vi "test-new-clock64-benchmark.vi"() -> ()   [LabVIEW 2020]
uses:
  <vilib>/Rock Robotics/WPI/ThirdParty/JAS_Junk/TrajLib/VI/Util_GetTime_U32.vi
  <vilib>/Rock Robotics/SystemInterfaces/Utilities/FPGA_UtilitiesRead LocalTime.vi
  <vilib>/Rock Robotics/WPI/ThirdParty/JAS_Junk/TrajLib/Trajectory_Library.lvlib
panel:
  out "Avg Loop US":dbl
  out "Per Loop US":dbl
  out "Error Count":i32
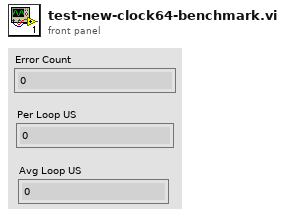
[diagram p1: front panel]
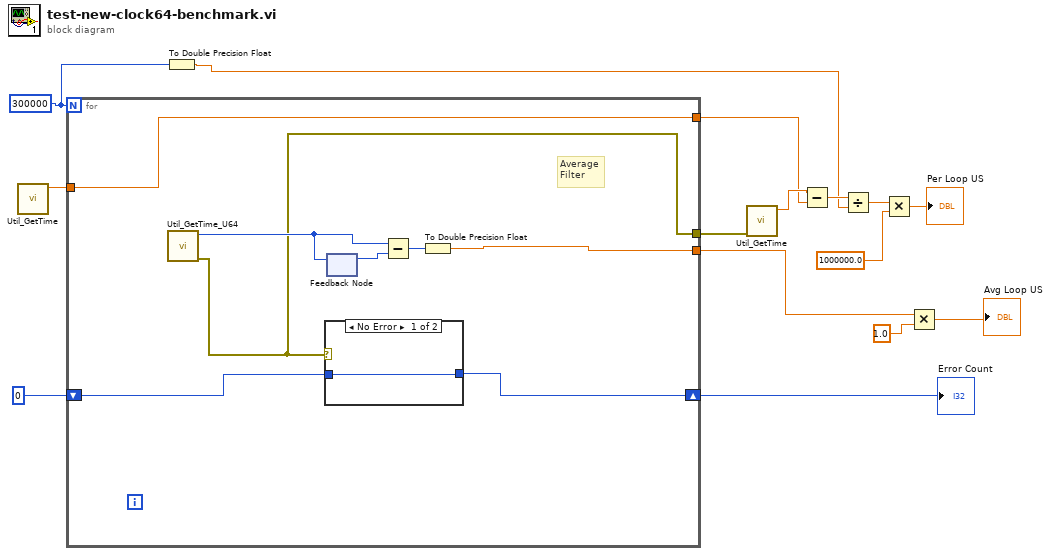
[diagram p0: block diagram]
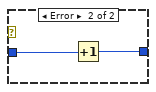
[diagram p2: hidden frame]
diagram:
  w13 = 300000
  n1 = call <vilib>:"Util_GetTime.vi"() -> ("FPGA_Time_Seconds"=w15:dbl)  [unwired: 8 in, 3 out]
  n2 = for {
    N: w13 -> [_]
    tunnel: w15 -> [w20]
    shift-right: [w21] -> w9
    shift-left: 0 -> [w23]
    tunnel: [w16] -> w4
    tunnel: [w20] -> w6
    tunnel: [w17] -> w2
    # "Average\nFilter"
    n3 = call <vilib>:"Util_GetTime_U64.vi"() -> ("error out"=w17:errorcluster, "FPGA_Time_MicroSeconds"=w19:u64)  [unwired: 10 in]
    n4 = case shown="No Error" w17 {
      tunnel: [w24 w26] -> w21
      tunnel: w23 -> [w24 w25]
      frame No Error {
      }
      frame Error {
        n5 = Increment(x=w25) -> (x+1=w26:i32)
      }
    }
    n6 = feedback-in #1(w19) -> ()
    n7 = feedback #1() -> (w22:u64)  [unwired: 1 in]
    n8 = Subtract(x=w19, y=w22) -> (x-y=w18:u64)
    n9 = To Double Precision Float(number=w18) -> (double precision float=w16:dbl)
  }
  "Error Count" <- w9
  n10 = To Double Precision Float(number=w13) -> (double precision float=w11:dbl)
  n11 = call <vilib>:"Util_GetTime.vi"("error in (no error)"=w2) -> ("FPGA_Time_Seconds"=w7:dbl)  [unwired: 7 in, 3 out]
  n12 = Subtract(x=w7, y=w6) -> (x-y=w12:dbl)
  n13 = Divide(x=w12, y=w11) -> (x/y=w10:dbl)
  n14 = Multiply(x=w10, y=1000000.0) -> (x*y=→"Per Loop US":dbl)
  n15 = Multiply(x=w4, y=1.0) -> (x*y=→"Avg Loop US":dbl)
